vi "Start.vi"(8 "error in (no error)":errorcluster, 11 "WaveSourceBlock in":refnum<class "WaveSourceBlock.lvclass">) -> (0 "error out":errorcluster, 3 "WaveSourceBlock out":refnum<class "WaveSourceBlock.lvclass">)   [LabVIEW 2020, in "WaveSourceBlock.lvclass"]
uses:
  WaveSourceBlock.lvclass
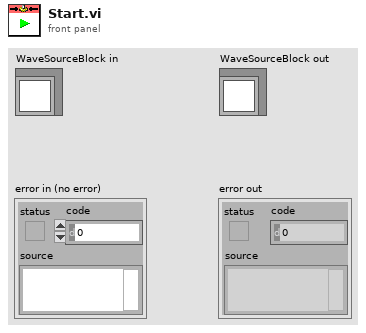
[diagram p1: front panel]
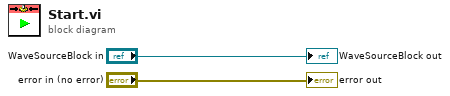
[diagram p0: block diagram]
diagram:
  "error out" <- "error in (no error)"
  "WaveSourceBlock out" <- "WaveSourceBlock in"
